vi "Tab_001_PH.vi"() -> ()   [LabVIEW 2021]
panel:
  out "Array 4":ext[][](array[numeric])=[[8.5, 11.8], [9.6000000000000000003, 12.9], [10.7, 14.1]]
  out "Array 2":i32[](array[numeric])=[0, 0, 0, 5, 6, 7]
  in  "Array":i32[](array[numeric])=[5, 6, 7, 5, 6, 7]
  in  "Array 3":ext[][](array[numeric])=[[8.5, 11.8], [9.6000000000000000003, 12.9], [10.7, 14.1]]
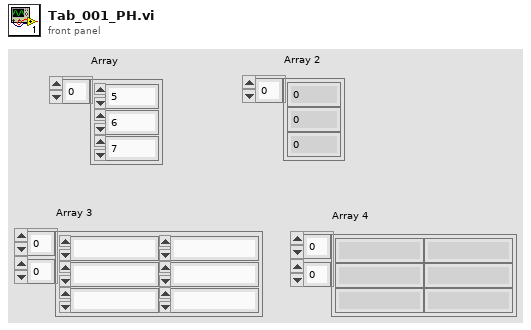
[diagram p1: front panel]
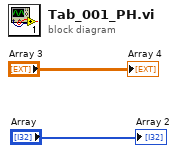
[diagram p0: block diagram]
diagram:
  "Array 2" <- "Array"
  "Array 4" <- "Array 3"
